vi "Create Listener.vi"(8 "error in (no error)":errorcluster, 9 "timeout ms (5000)":i32=5000, 10 "Port":u16, 11 "Socket Listener in":refnum<class "Socket Listener.lvclass">) -> (0 "error out":errorcluster, 3 "Socket Listener out":refnum<class "Socket Listener.lvclass">)   [LabVIEW 2021, in "Sockets.lvlib" / "Socket Listener.lvclass"]
doc: "Creates a new TCP listener on the requested port.\nWebSockets 2.0.1.40\nSam Sharp - MediaMongrels Ltd\nCopyright (c) 2019, MediaMongrels Ltd"
uses:
  Socket Listener.lvclass
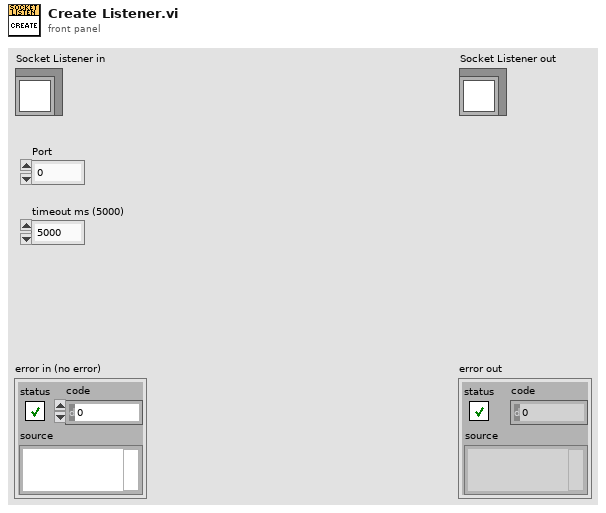
[diagram p1: front panel]
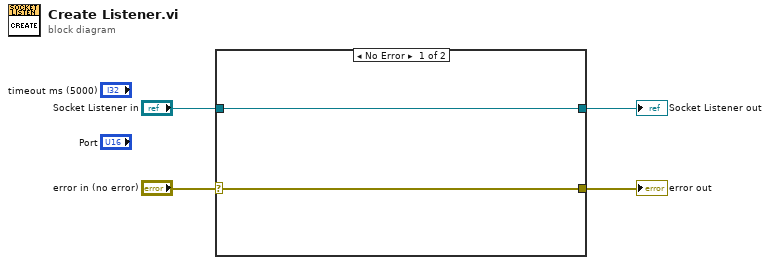
[diagram p0: block diagram]
diagram:
  n1 = case shown="No Error" "error in (no error)" {
    selector: "error in (no error)" -> [w5 w8]
    tunnel: [w5 w8] -> w3
    tunnel: [w6 w7] -> w1
    tunnel: "Socket Listener in" -> [w6 w7]
    frame No Error {
    }
    frame Error {
    }
  }
  "error out" <- w3
  "Socket Listener out" <- w1
